vi "Read Multi Eval Meas SEM Results.vi"(8 "error in (no error)":errorcluster, 9 "Result Type (Current)":i32(ring) items=["Current", "Average", "Extreme", "Standard Deviation"], 10 "Instance (1)":T2=1, 11 "VISA resource name":refnum<visa-resource-name>) -> (0 "error out":errorcluster, 1 "SEM Results":T1 {"TX Power" format="%^.3e"; "OBW" format="%^.3e"; "Out Of Tolerance" format="%^.3e"}, 2 "Reliability":i32, 3 "VISA resource name out":refnum<visa-resource-name>)   [LabVIEW 2015, in "Rohde&Schwarz CMXP NR FR2 Measurement.lvlib"]
doc: "Starts a new single shot measurement and returns the average value results of the spectrum emission measurement.\n\nAttributes:\nRSCMXPNRFR2M_ATTR_READ_MULTI_EVAL_MEASUREMENT_SEM_AVERAGE_RESULTS\nRSCMXPNRFR2M_ATTR_READ_MULTI_EVAL_MEASUREMENT_SEM_CURRENT_RESULTS\nRSCMXPNRFR2M_ATTR_READ_MULTI_EVAL_MEASUREMENT_SEM_STANDARD_DEVIATION_RESULTS\nRSCMXPNRFR2M_ATTR_READ_MULTI_EVAL_MEASUREMENT_SEM_EXTREME_RESULTS\n\nRemote-control commands:\nREAD:NRMMw:MEAS<i>:MEValuation:SEMask:AVERage?\nREAD:NRMMw:MEAS<i>:MEValuation:SEMask:CURRent?\nREAD:NRMMw:MEAS<i>:MEValuation:SEMask:SDEViation?"
uses:
  <instrlib>/Rohde&Schwarz CMXP NR FR2 Measurement/Rohde&Schwarz CMXP NR FR2 Measurement.lvlib
  <instrlib>/Rohde&Schwarz CMXP NR FR2 Measurement/Private/_Instance.ctl
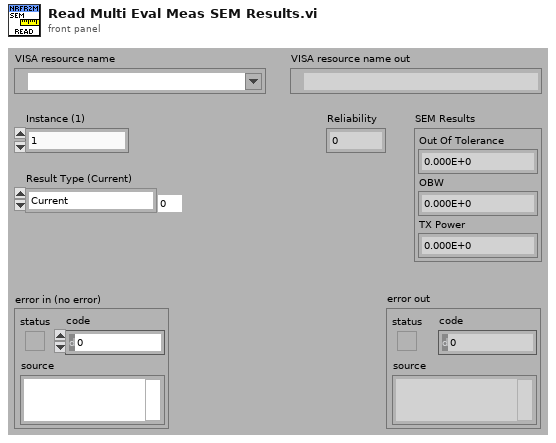
[diagram p1: front panel]
types:
  T1 = cluster{"Out Of Tolerance":dbl, "OBW":dbl, "TX Power":dbl}
  T2 = typedef "Rohde&Schwarz CMXP NR FR2 Measurement.lvlib/_Instance.ctl" = i32
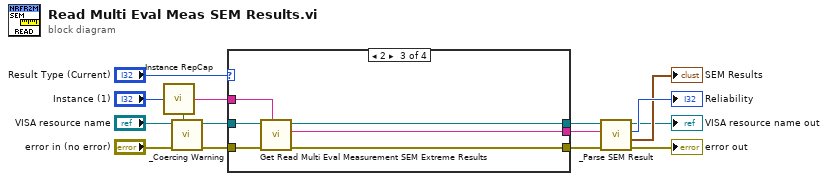
[diagram p0: block diagram]
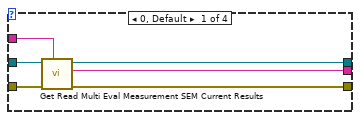
[diagram p2: hidden frame]
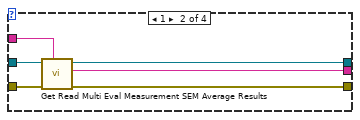
[diagram p3: hidden frame]
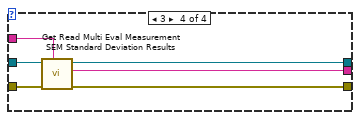
[diagram p4: hidden frame]
diagram:
  n1 = call <instrlib>:"Instance RepCap.vi"("Instance In"="Instance (1)") -> ("In Range?"=w13:bool, "RepCap Identifier Out"=w10:string)  [unwired: 1 in]
  n2 = call <instrlib>:"_Coercing Warning.vi"("In Range?"=w13, "error in (no error)"="error in (no error)", "VISA resource name"="VISA resource name") -> ("error out"=w12:errorcluster, "VISA resource name out"=w11:refnum<visa-resource-name>)  [unwired: 7 in]
  n3 = case shown="2" "Result Type (Current)" {
    tunnel: w12 -> [w21 w27 w33 w39]
    tunnel: w11 -> [w20 w26 w32 w38]
    tunnel: w10 -> [w19 w25 w31 w37]
    tunnel: [w18 w24 w30 w34] -> w8
    tunnel: [w17 w23 w29 w36] -> w7
    tunnel: [w16 w22 w28 w35] -> w6
    frame 0, Default {
      n4 = call "Get Read Multi Eval Measurement SEM Current Results"("Repeated Capabilities"=w19, "error in (no error)"=w21, "instrument handle"=w20) -> ("error out"=w18:errorcluster, "Read Multi Eval Measurement SEM Current Results"=w16:string, "instrument handle out"=w17:refnum<visa-resource-name>)  [unwired: 6 in]
    }
    frame 1 {
      n5 = call "Get Read Multi Eval Measurement SEM Average Results"("Repeated Capabilities"=w25, "error in (no error)"=w27, "instrument handle"=w26) -> ("error out"=w24:errorcluster, "Read Multi Eval Measurement SEM Average Results"=w22:string, "instrument handle out"=w23:refnum<visa-resource-name>)  [unwired: 6 in]
    }
    frame 2 {
      n6 = call "Get Read Multi Eval Measurement SEM Extreme Results"("Repeated Capabilities"=w31, "error in (no error)"=w33, "instrument handle"=w32) -> ("error out"=w30:errorcluster, "Read Multi Eval Measurement SEM Extreme Results"=w28:string, "instrument handle out"=w29:refnum<visa-resource-name>)  [unwired: 6 in]
    }
    frame 3 {
      n7 = call "Get Read Multi Eval Measurement SEM Standard Deviation Results"("Repeated Capabilities"=w37, "error in (no error)"=w39, "instrument handle"=w38) -> ("error out"=w34:errorcluster, "Read Multi Eval Measurement SEM Standard Deviation Results"=w35:string, "instrument handle out"=w36:refnum<visa-resource-name>)  [unwired: 6 in]
    }
  }
  n8 = call <instrlib>:"_Parse SEM Result.vi"("error in (no error)"=w8, "Input String"=w6, "VISA resource name"=w7) -> ("error out"=→"error out":errorcluster, "Measurement Result"=→"SEM Results":T1, "Reliability"=→"Reliability":i32, "VISA resource name out"=→"VISA resource name out":refnum<visa-resource-name>)  [unwired: 5 in]
